vi "Example Diagram Constants.vi"(8 "Error In":errorcluster) -> (0 "Error Out":errorcluster)   [LabVIEW 2014]
uses:
  <vilib>/measure/NI_MABase.lvlib
panel:
  out "x+y":i32
  out "numeric const. FXP 1":fxp<+,1,1>
  out "lubo string const. ABC":string="42 hello world!"
  out "numeric const. B":i32
  out "numeric const. A":i32
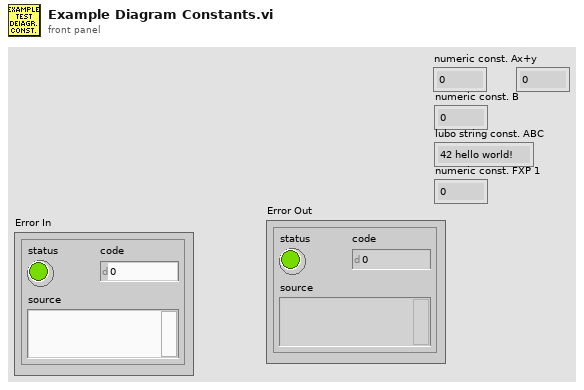
[diagram p1: front panel]
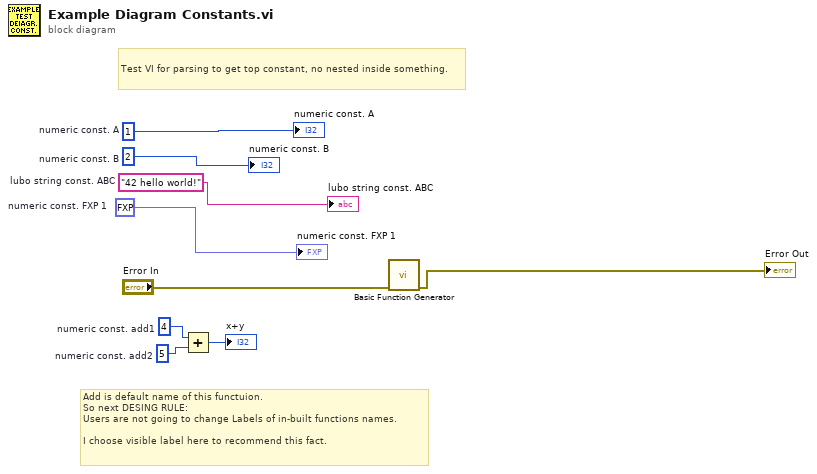
[diagram p0: block diagram]
diagram:
  w3 = 5  # numeric const. add2
  w2 = 4  # numeric const. add1
  w7 = "42 hello world!"  # lubo string const. ABC
  w6 = fxp<+,2,2> 3.0  # numeric const. FXP 1
  w8 = 2  # numeric const. B
  w9 = 1  # numeric const. A
  # "Add is default name of this functuion.\nSo next DESING RULE:\nUsers are not going to change Labels of in-built functions names.\n\nI choose visible label here to recommend this fact."
  # "Test VI for parsing to get top constant, no nested inside something."
  n1 = Add(x=w2, y=w3) -> (x+y=→"x+y":i32)
  n2 = call <vilib>:"Basic Function Generator.vi"("error in (no error)"="Error In") -> ("error out"=→"Error Out":errorcluster)  [unwired: 8 in, 2 out]
  "numeric const. A" <- w9
  "numeric const. B" <- w8
  "lubo string const. ABC" <- w7
  "numeric const. FXP 1" <- w6
